vi "GetAppMetadataProperty.vi"(8 "No Error":errorcluster, 11 "Name":T1) -> (0 "error out":errorcluster, 2 "Found or Default":bool, 3 "Value or Default":string)   [LabVIEW 2026, in "SDL3.lvlib" / "Init.lvlib"]
doc: "<B>Summary</B>\nGet metadata about your app.\n\n<B>Remarks</B>\nThis returns metadata previously set using <B>SDL_SetAppMetadata()</B> or <B>SDL_SetAppMetadataProperty()</B>. See <B>SDL_SetAppMetadataProperty()</B> for the list of available properties and their meanings."
uses:
  Init.lvlib
  MetadataPropertyName--combobox.ctl
  Stdinc/Strlen.vi
  Stdinc/Strlen.vi/c3f57b18-2899-4d18-8de7-ed42e0d99649.vi
  <vilib>/Utility/error.llb/Error Cluster From Error Code.vi
  LV-Utilities/LV-Utilities.lvlib
  Lib/SDL3.dll
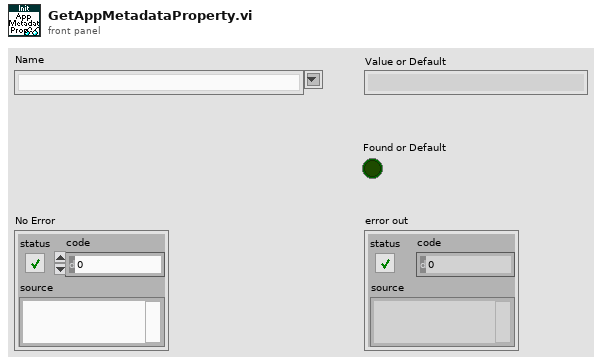
[diagram p1: front panel]
types:
  T1 = typedef "SDL3.lvlib/Init.lvlib/MetadataPropertyName--combobox.ctl" = string
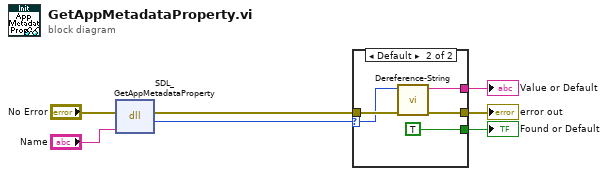
[diagram p0: block diagram]
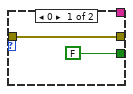
[diagram p2: hidden frame]
diagram:
  n1 = dll-call lib="C:/Users/saukko/Dev/LV-SDL3/Sources/SDL3/Lib/SDL3.*" fn="SDL_GetAppMetadataProperty"(error in="No Error", "name"="Name") -> (error out=w6:errorcluster, "return type"=w3:i64)  [unwired: 3 in, 1 out]
  n2 = case shown="Default" w3 {
    selector: w3 -> [_ w12]
    tunnel: w6 -> [w9 w14]
    tunnel: [w9 w13] -> w4
    tunnel: [_ w11] -> w2
    tunnel: [FALSE TRUE] -> w1
    frame 0 {
    }
    frame Default {
      n3 = call "Dereference-String.vi"("No Error"=w14, "Str [const char *]"=w12) -> ("error out"=w13:errorcluster, "String"=w11:string)  [unwired: 8 in]
    }
  }
  "error out" <- w4
  "Value or Default" <- w2
  "Found or Default" <- w1
